vi "binary_lights.vi"() -> ()   [LabVIEW 2016]
panel:
  out "Decimal":dbl
  in  "Binary Array":bool[](array[boolean])
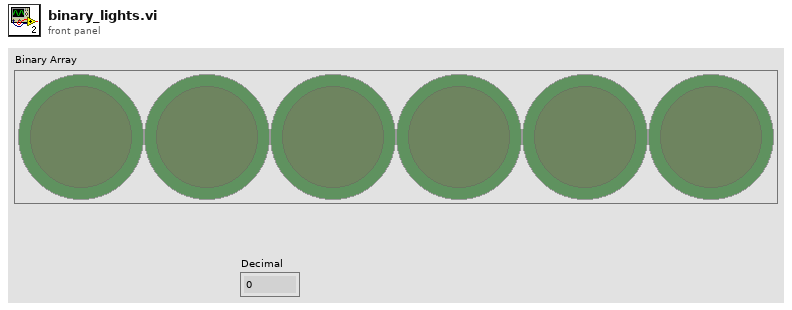
[diagram p1: front panel]
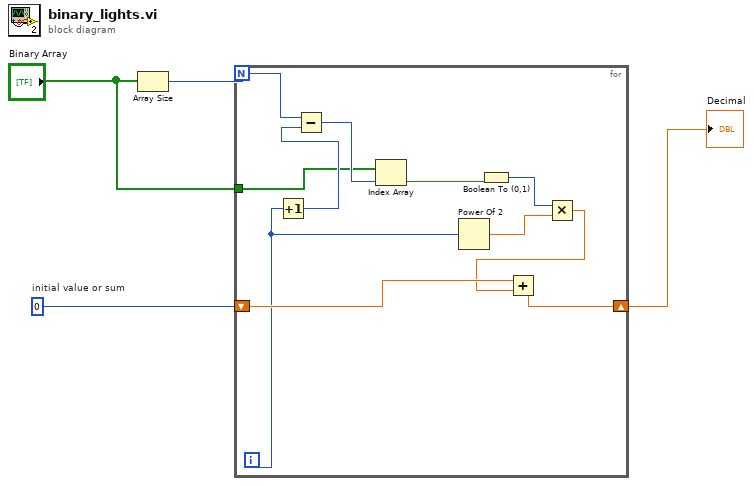
[diagram p0: block diagram]
diagram:
  w2 = 0  # initial value or sum
  n1 = Array Size(array="Binary Array") -> (size(s)=w4:i32)
  n2 = for {
    N: w4 -> [w14]
    tunnel: "Binary Array" -> [w11]
    shift-right: [w6] -> w1
    shift-left: w2 -> [w15]
    i -> [w9]
    n3 = Increment(x=w9) -> (x+1=w13:i32)
    n4 = Subtract(x=w14, y=w13) -> (x-y=w12:i32)
    n5 = Index Array(array=w11, index=w12) -> (element=w10:bool)
    n6 = Power Of 2(x=w9) -> (2^x=w7:dbl)
    n7 = Boolean To (0,1)(Boolean=w10) -> (0, 1=w8:i16)
    n8 = Multiply(x=w8, y=w7) -> (x*y=w5:dbl)
    n9 = Add(x=w15, y=w5) -> (x+y=w6:dbl)
  }
  "Decimal" <- w1
